vi "Dashboard Main.vi"() -> ()   [LabVIEW 2013]
uses:
  <vilib>/event_ctls.llb/eventvkey.ctl
panel:
  out "Encoder Speed":dbl(graph)
  in  "Rec Mode":enum32{"Stop", "Record", "Playback"}(radio)
  out "Battery":sgl
  out "High Gear":bool
  out "Speed":dbl(knob) scale=0.0..25.0
  out "Dashboard Connected":bool
  in  "Tab Control":enum32{"Auto", "Constants", "Checklist", "Gyro"}(tab)
  in  "Autonmous To Run":string(combo)
  in  "Autonmous mode":string
  in  "Editable":bool
  in  "Reload Autonmous text file":bool
  in  "Save Auto file back to text file":bool
  in  "Reload Constants":bool
  out "Variable Names":string[](array[string])
  out "Array of Numbers":dbl[](array[numeric])
  in  "Listbox":i32(listbox)
  in  "Reset Gyro":bool
  out "gyroAngle":dbl
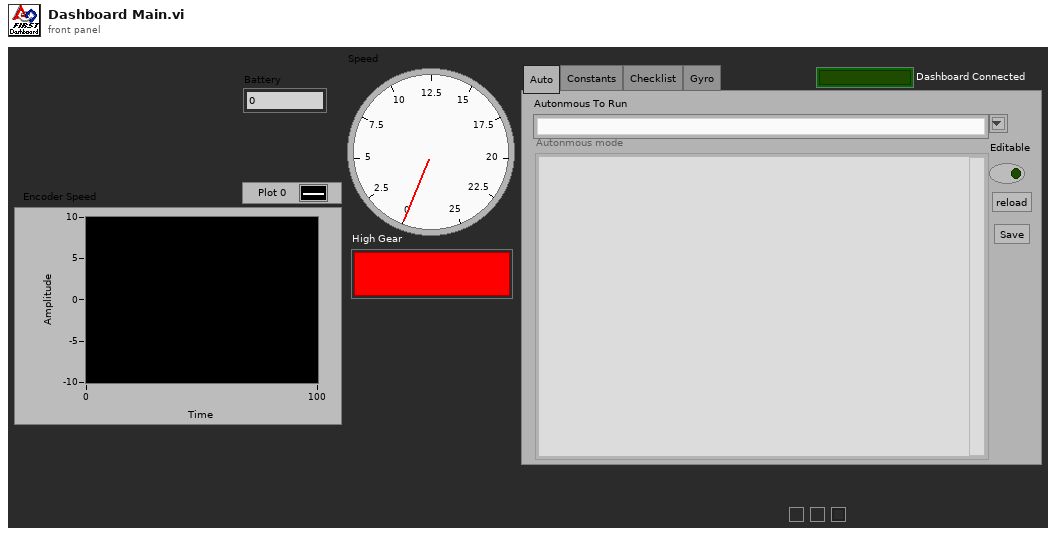
[diagram p1: front panel]
types:
  T1 = enum16{"None", "On Hover", "On Key Focus", "On Hover or Key Focus"}
  T2 = enum8{"Enabled", "Disabled", "Disabled and Grayed Out"}
  T3 = cluster{"Digital Inputs":bool[], "Digital Outputs":bool[]}
  T4 = cluster{"Competition mode":bool, "Robot Link":bool, "Autonomous":bool, "Enabled":bool, "E-Stop":bool, "Simulated":bool, "TestMode":bool, "Docked Window":bool}
  T5 = typedef "eventvkey.ctl" = enum16{"ASCII", "Enter", "Return", "Shift", "Ctrl", "Alt", "Cmd", "Opt", "Caps", "NumLock", "Clear", "Break", "Up", "Down", "Left", "Right", "Insert", "Delete", "Home", "End", "PageUp", "PageDown", "Escape", "Help", "Pause", "ScrollLock", "F1", "F2", "F3", "F4", "F5", "F6", "F7", "F8", "F9", "F10", "F11", "F12", "F13", "F14", "F15", "F16", "F17", "F18", "F19", "F20", "F21", "F22", "F23", "F24", "Play", "VolumeUp", "VolumeDown", "Mute", "Two Byte Char"}
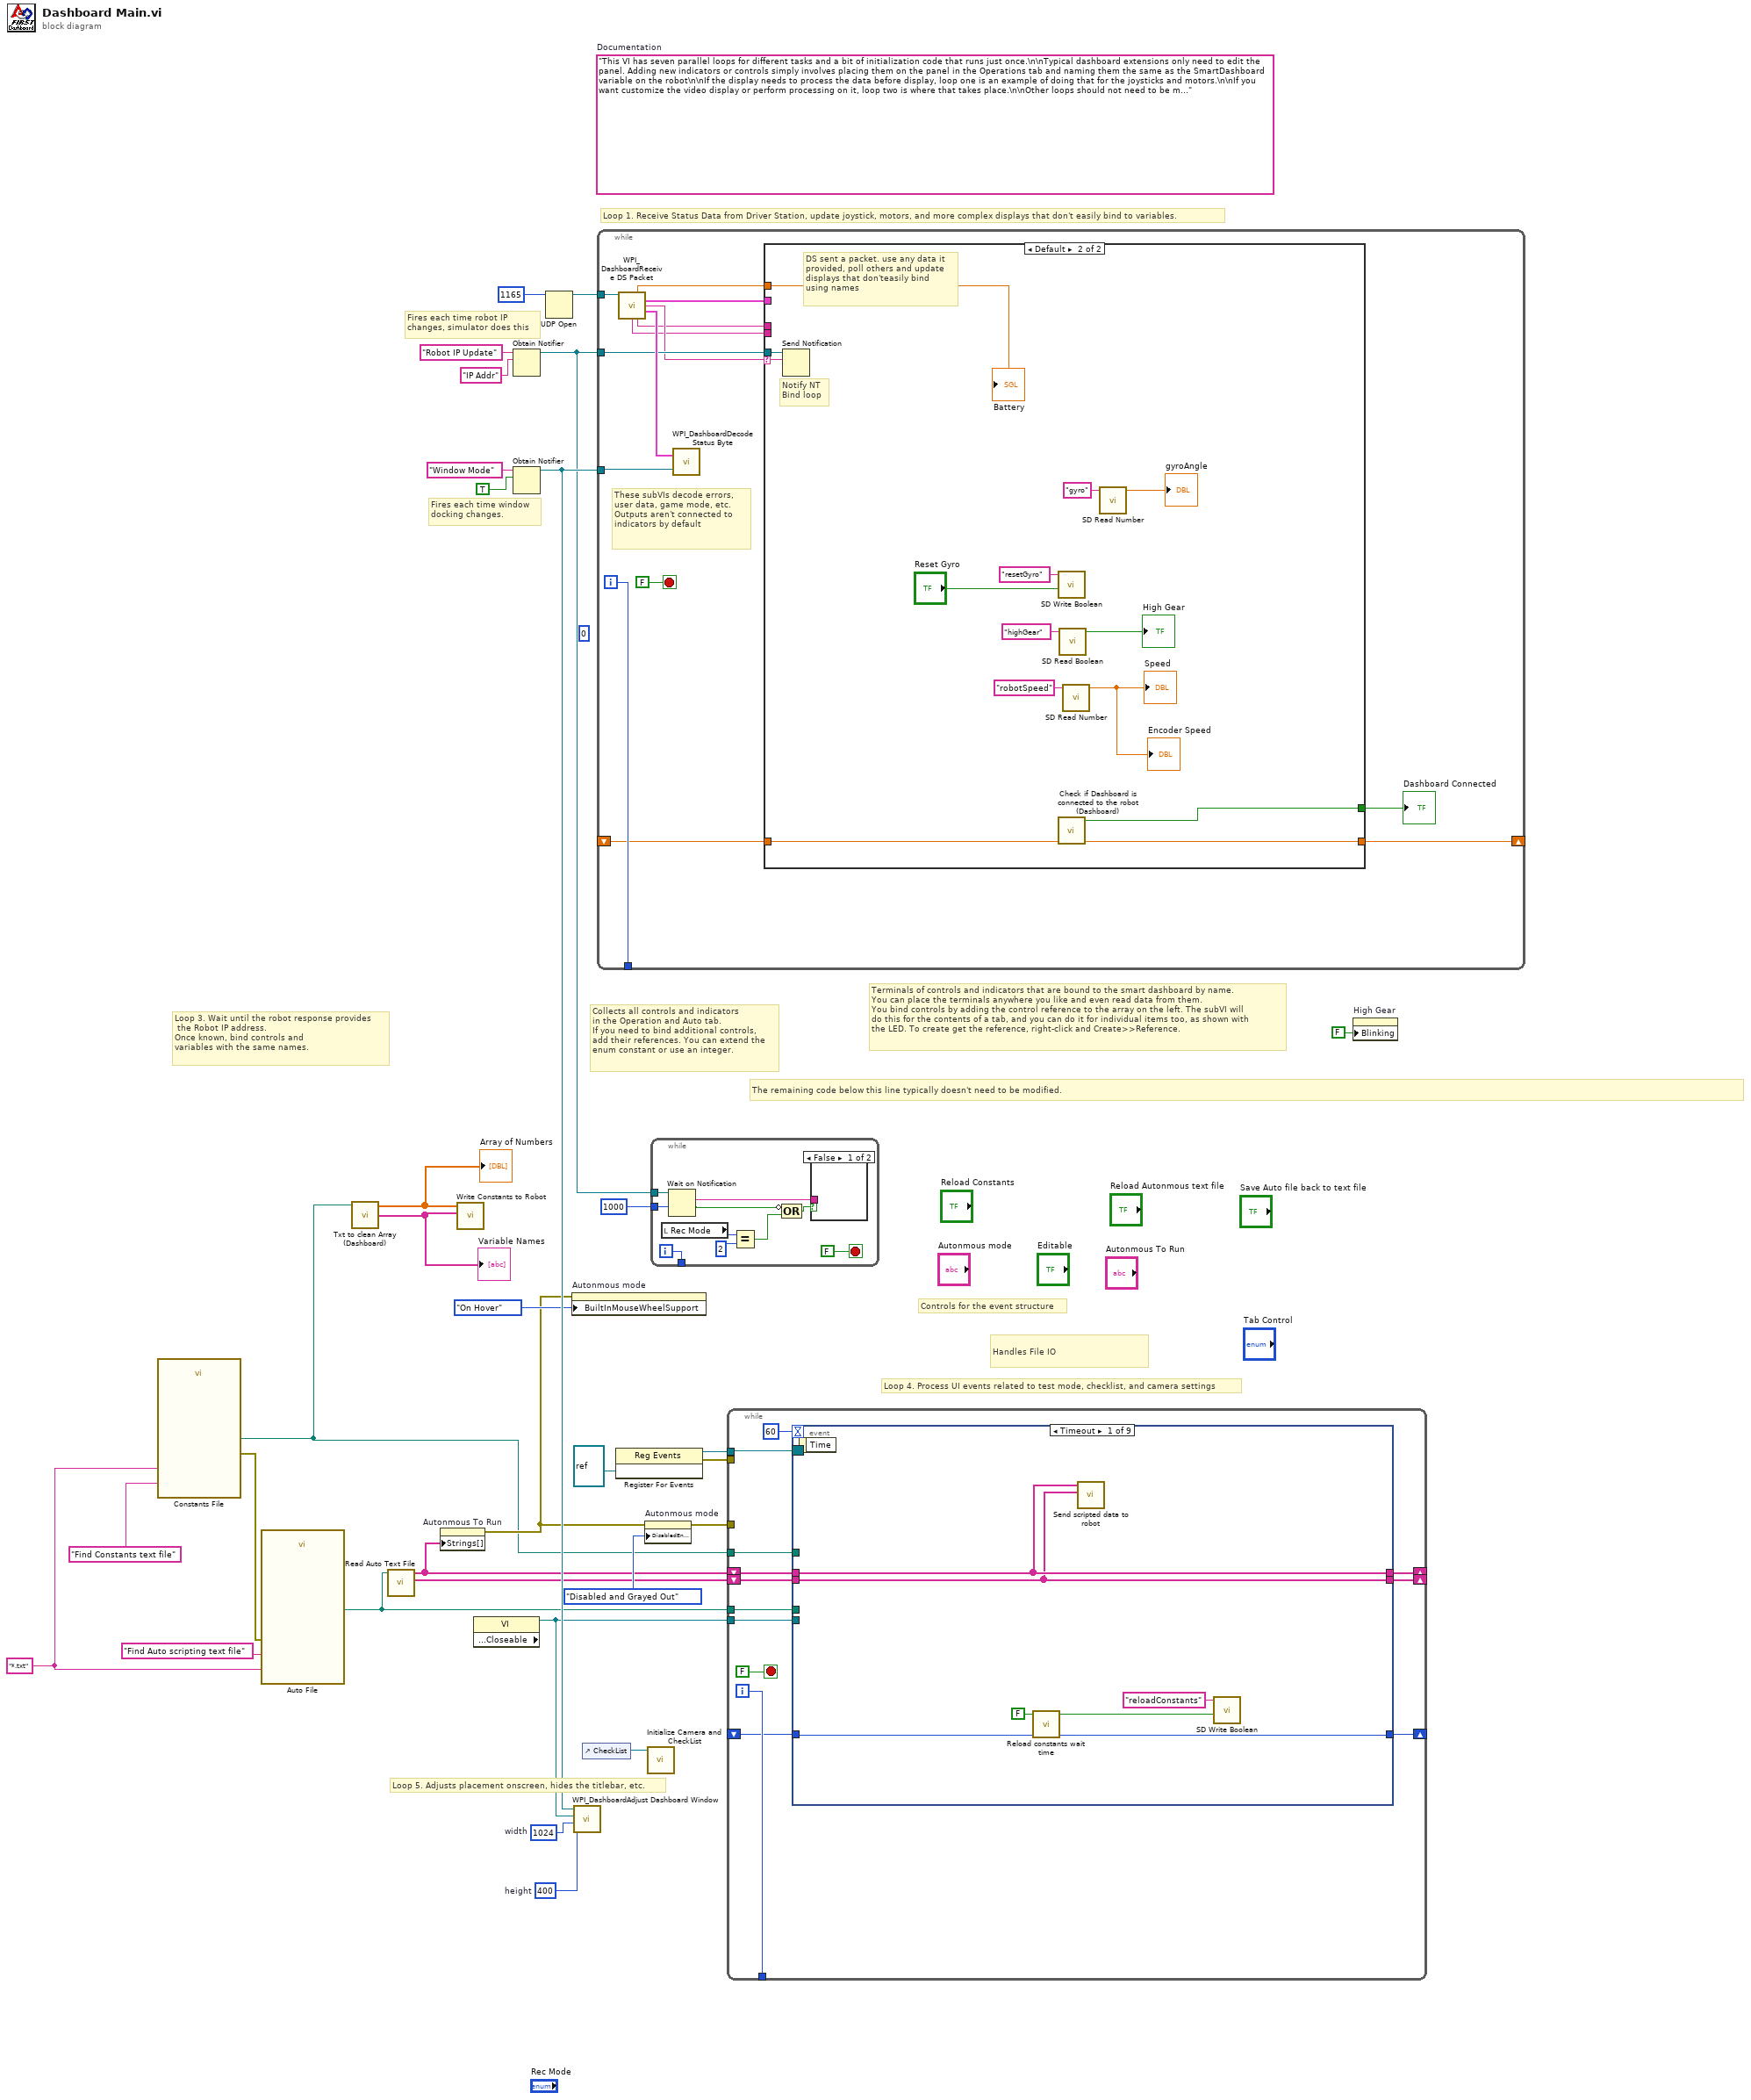
[diagram p0: block diagram]
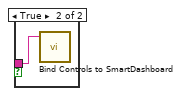
[diagram p2: hidden frame]
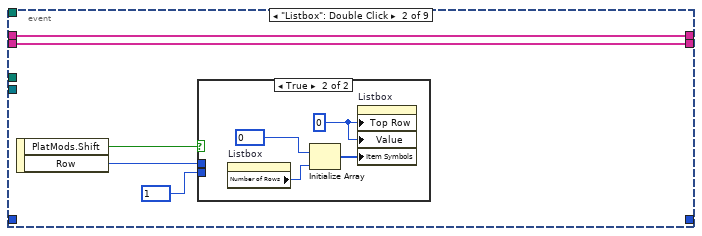
[diagram p3: hidden frame]
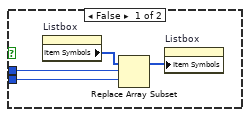
[diagram p4: hidden frame]
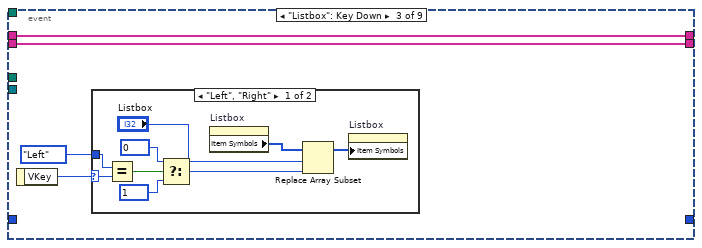
[diagram p5: hidden frame]
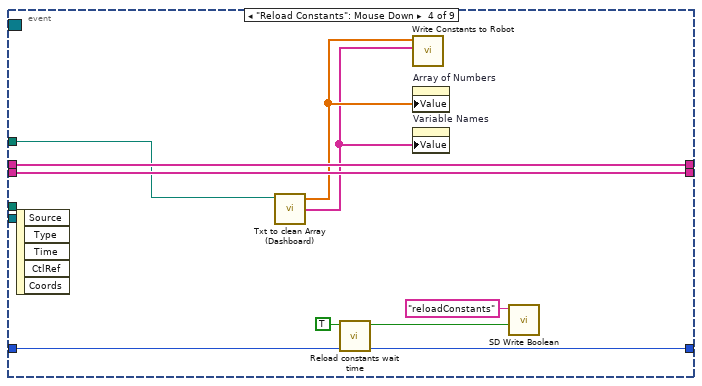
[diagram p7: hidden frame]
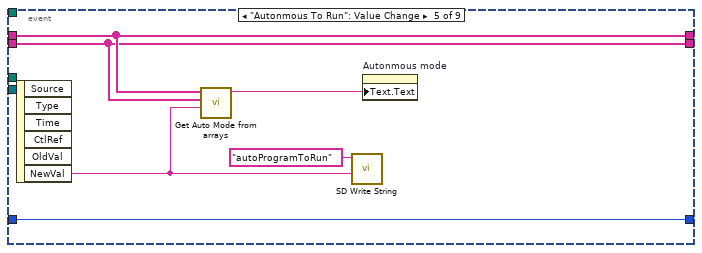
[diagram p8: hidden frame]
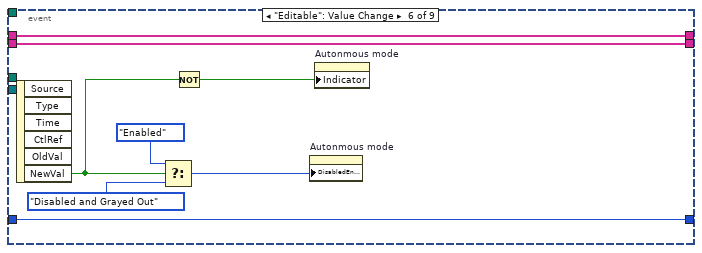
[diagram p9: hidden frame]
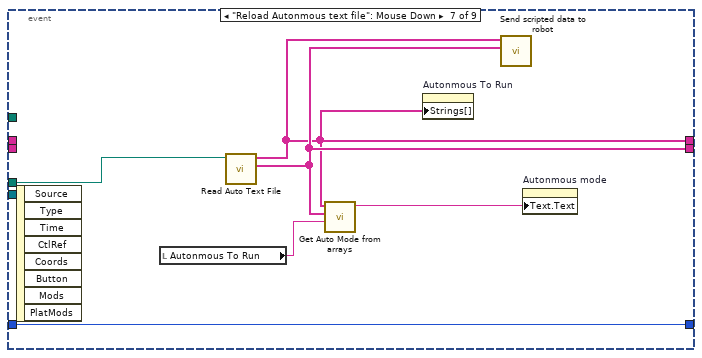
[diagram p10: hidden frame]
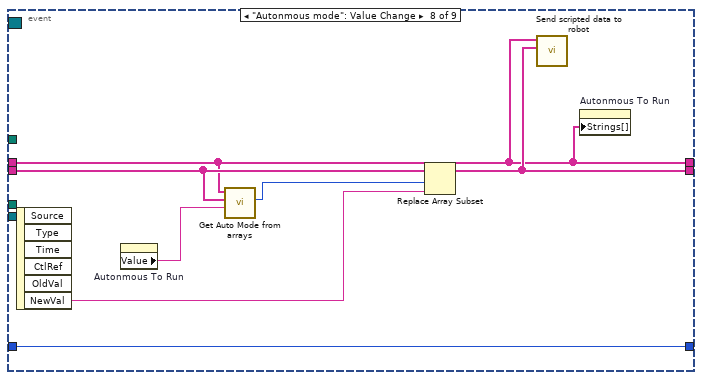
[diagram p11: hidden frame]
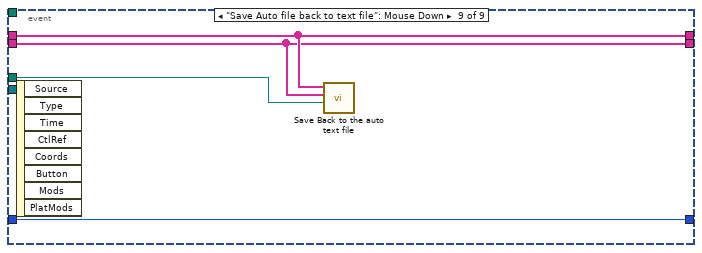
[diagram p12: hidden frame]
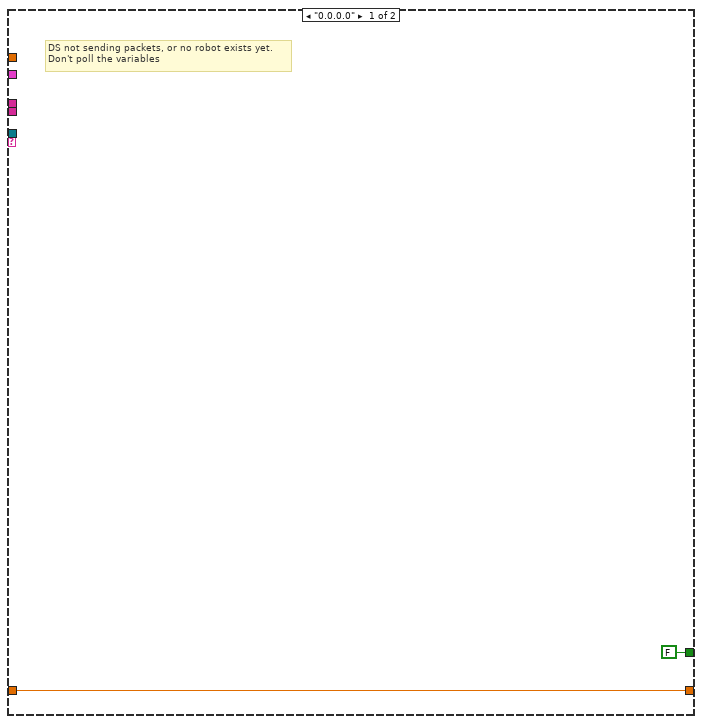
[diagram p13: hidden frame]
diagram:
  (unwired) u32 0 ("millisecond timer value out")
  w7 = "*.txt" ("pattern label")
  w21 = 400  # height
  w22 = 1024  # width
  (unwired) "This VI has seven parallel loops for different tasks and a bit of initialization code that runs just once.\n\nTypical dashboard extensions only need to edit the panel. Adding new indicators or controls simply involves placing them on the panel in the Operations tab and naming them the same as the SmartDashboard variable on the robot\n\nIf the display needs to process the data before display, loop one is an example of doing that for the joysticks and motors.\n\nIf you want customize the video display or perform processing on it, loop two is where that takes place.\n\nOther loops should not need to be modified. They are pretty standard, and document the task they perform."  # Documentation
  # "Loop 3. Wait until the robot response provides\n the Robot IP address.\nOnce known, bind controls and\nvariables with the same names."
  # "Controls for the event structure"
  # "Handles File IO"
  # "Fires each time robot IP\nchanges, simulator does this"
  # "Fires each time window\ndocking changes."
  # "Collects all controls and indicators\nin the Operation and Auto tab.\nIf you need to bind additional controls,\nadd their references. You can extend the\nenum constant or use an integer."
  # "The remaining code below this line typically doesn't need to be modified."
  # "Loop 4. Process UI events related to test mode, checklist, and camera settings"
  # "Terminals of controls and indicators that are bound to the smart dashboard by name.\nYou can place the terminals anywhere you like and even read data from them.\nYou bind controls by adding the control reference to the array on the left. The subVI will\ndo this for the contents of a tab, and you can do it for individual items too, as shown with\nthe LED. To create get the reference, right-click and Create>>Reference."
  # "Loop 5. Adjusts placement onscreen, hides the titlebar, etc."
  # "Loop 1. Receive Status Data from Driver Station, update joystick, motors, and more complex displays that don't easily bind to variables."
  n1 = call "Constants File"("prompt"="Find Constants text file", "pattern (all files)"=w7) -> ("selected path"=w10:path, "error out"=w9:errorcluster)  [unwired: 10 in, 2 out]
  n2 = call "Auto File"("prompt"="Find Auto scripting text file", "error in"=w9, "pattern (all files)"=w7) -> ("selected path"=w17:path)  [unwired: 9 in, 3 out]
  n3 = call "Txt to clean Array (Dashboard).vi"("file path"=w10) -> ("Variable Names"=w4:string[], "Array of Numbers"=w5:dbl[])  [unwired: 3 in, 1 out]
  "Array of Numbers" <- w5
  "Variable Names" <- w4
  n4 = call "Read Auto Text File.vi"("selected path"=w17) -> ("Programs"=w14:string[], "Program Name"=w15:string[])  [unwired: 8 in, 1 out]
  n5 = property on="Autonmous To Run" class="CmbBox"("Strings[]"=w15) -> (error out=w12:errorcluster)  [unwired: 2 in, 1 out]
  n6 = call "Write Constants to Robot.vi"("Variable Names"=w4, "Array of Numbers"=w5) -> ()  [unwired: 10 in]
  n7 = property class="VI" props=["Front Panel.Closeable"]() -> (reference out=w18:refnum<vi>)  [unwired: 2 in, 2 out]
  n8 = Obtain Notifier(name (unnamed)="Robot IP Update", notification data type="IP Addr" ("name (unnamed)")) -> (notifier out=w1:refnum<notifier>)  [unwired: 2 in, 2 out]
  n9 = Obtain Notifier(name (unnamed)="Window Mode", notification data type=TRUE) -> (notifier out=w20:refnum<notifier>)  [unwired: 2 in, 2 out]
  n10 = UDP Open(11:u16 1165 ("port")) -> (port=w30:refnum<k16>)  [unwired: 2 in, 4 out]
  n11 = property on="Autonmous mode" class="Str"(error in=w12, "BuiltInMouseWheelSupport"=T1."On Hover" ("Built-In Mouse Wheel Support")) -> ()  [unwired: 1 in, 2 out]
  n12 = call <vilib>:"WPI_DashboardAdjust Dashboard Window.vi"("height"=w21, "width"=w22, "reference in"=w18, "Notifier in"=w20) -> ()  [unwired: 8 in]
  n13 = control-ref of="CheckList"() -> (w19:refnum<vi>)
  n14 = while {
    tunnel: w30 -> [w43]
    tunnel: w1 -> [w40]
    tunnel: w20 -> [w42]
    tunnel: [w41] -> _
    shift-right: [w34] -> _
    shift-left: _ -> [w33]
    i -> [w41]
    stop <- FALSE stop-if-true
    # "These subVIs decode errors, user data, game mode, etc.\nOutputs aren't connected to indicators by default"
    n15 = call <vilib>:"WPI_DashboardReceive DS Packet.vi"("Recv Socket"=w43) -> ("Battery"=w35:sgl, "Driver Station"=w36:T3, "Robot IP Address"=w39:string, "Status"=w44:T4, "Low Priority User Data"=w38:string, "High Priority User Data"=w37:string)  [unwired: 1 in, 8 out]
    n16 = call <vilib>:"WPI_DashboardDecode Status Byte.vi"("Window Mode Notifier"=w42, "Status"=w44) -> ()  [unwired: 2 out]
    n17 = case shown="Default" w39 {
      selector: w39 -> [_ w60]
      tunnel: w40 -> [_ w61]
      tunnel: w38 -> [_ _]
      tunnel: w37 -> [_ _]
      tunnel: w36 -> [_ _]
      tunnel: w35 -> [_ w54]
      tunnel: [w47 w59] -> w34
      tunnel: w33 -> [w47 w58]
      tunnel: [FALSE ("Number Changing") w53] -> w32
      frame "0.0.0.0" {
        # "DS not sending packets, or no robot exists yet.\nDon't poll the variables"
      }
      frame Default {
        # "Notify NT\nBind loop"
        # "DS sent a packet. use any data it\nprovided, poll others and update\ndisplays that don'teasily bind\nusing names"
        n18 = Send Notification(notification=w60, notifier=w61) -> ()  [unwired: 1 in, 2 out]
        n19 = call <vilib>:"SD Write Boolean.vi"("Boolean"="Reset Gyro", "Name"="resetGyro") -> ()  [unwired: 8 in, 2 out]
        n20 = call "Check if Dashboard is connected to the robot (Dashboard).vi"("From shift"=w58) -> ("to shift"=w59:dbl, "Number Changing"=w53:bool)  [unwired: 9 in]
        n21 = call <vilib>:"SD Read Boolean.vi"("Name"="highGear") -> ("Boolean"=→"High Gear":bool)  [unwired: 8 in, 2 out]
        n22 = call <vilib>:"SD Read Number.vi"("Name"="robotSpeed") -> ("Numeric"=→"Speed" →"Encoder Speed":dbl)  [unwired: 8 in, 2 out]
        n23 = call <vilib>:"SD Read Number.vi"("Name"="gyro") -> ("Numeric"=→"gyroAngle":dbl)  [unwired: 8 in, 2 out]
        "Battery" <- w54
      }
    }
    "Dashboard Connected" <- w32
  }
  n24 = register-events(refnum<vi> refnum) -> (reference out=w25:refnum<event-registration>, error out=w24:errorcluster)  [unwired: 2 in]
  n25 = property on="Autonmous mode" class="Str"(error in=w12, "DisabledEnum"=T2."Disabled and Grayed Out" ("Disabled")) -> (error out=w11:errorcluster)  [unwired: 1 in, 1 out]
  n26 = call "Initialize Camera and CheckList.vi"("ListBox in"=w19) -> ()  [unwired: 11 in]
  n27 = while {
    tunnel: w1 -> [w70]
    tunnel: [w68] -> _
    tunnel: u32 1000 ("milliseconds to wait") -> [w67]
    i -> [w68]
    stop <- FALSE stop-if-true
    n28 = local read "Rec Mode"() -> (w63:enum32{"Stop", "Record", "Playback"})
    n29 = Wait on Notification(notifier=w70, timeout in ms (-1)=w67) -> (notification=w69:string, timed out?=w65:bool)  [unwired: 2 in, 2 out]
    n30 = Equal?(x=w63, y=u16 2 ("Rec Mode")) -> (x = y?=w64:bool)
    n31 = Compound Arithmetic op=OR(invert w65, w64) -> (w66:bool)
    n32 = case shown="False" w66 {
      tunnel: w69 -> [_ w72]
      frame False {
      }
      frame True {
        n33 = call <vilib>:"Bind Controls to SmartDashboard.vi"("Server IP Address"=w72) -> ()  [unwired: 11 in]
      }
    }
  }
  n34 = while {
    tunnel: [w83] -> _
    tunnel: w25 -> [w82]
    tunnel: w24 -> [_]
    tunnel: w18 -> [w81]
    tunnel: w17 -> [w80]
    tunnel: w10 -> [w79]
    shift-right: [w76] -> _
    shift-left: w15 -> [w78]
    shift-right: [w75] -> _
    shift-left: w14 -> [w77]
    tunnel: w11 -> [_]
    shift-right: [w74] -> _
    shift-left: _ -> [w73]
    i -> [w83]
    stop <- FALSE stop-if-true
    n35 = event shown="[0] Timeout" {
      selector: w82 -> [_ _ _ _ _ _ _ _ _]
      dyn-events: _ -> [_ _ _ _ _ _ _ _ _]
      timeout: u32 60 ("milliseconds to wait") -> [_ _ _ _ _ _ _ _ _]
      tunnel: w81 -> [_ _ _ _ _ _ _ _ _]
      tunnel: w80 -> [_ _ _ _ _ _ w148 _ w157]
      tunnel: w79 -> [_ _ _ w126 _ _ _ _ _]
      tunnel: w77 -> [w91 w93 w106 w127 w130 w136 _ w154 w158]
      tunnel: w78 -> [w92 w94 w107 w128 w131 w137 _ w151 w159]
      tunnel: [w92 w94 w107 w128 w131 w137 w144 w151 w159] -> w76
      tunnel: [w91 w93 w106 w127 w130 w136 w147 w152 w158] -> w75
      tunnel: [w89 _ _ w122 w129 w135 w143 w149 w156] -> w74
      tunnel: w73 -> [w90 _ _ w123 w129 w135 w143 w149 w156]
      event Timeout {
        n36 = event-data() -> ()  [unwired: 1 in, 1 out]
        n37 = call "Reload constants wait time.vi"("millisecond timer value in"=w90, "Reload Constants"=FALSE) -> ("millisecond timer value out"=w89:u32, "Tell Robot to reload constants"=w86:bool)  [unwired: 8 in]
        n38 = call "Send scripted data to robot.vi"("Programs"=w91, "Program Name"=w92) -> ()  [unwired: 10 in]
        n39 = call <vilib>:"SD Write Boolean.vi"("Boolean"=w86, "Name"="reloadConstants") -> ()  [unwired: 8 in, 2 out]
      }
      event "Listbox": Double Click {
        n40 = event-data() -> ("PlatMods.Shift"=w95:bool, "Row"=w97:i32)  [unwired: 1 in]
        n41 = case shown="True" w95 {
          tunnel: w97 -> [w101 _]
          tunnel: 1 -> [w100 _]
          frame False {
            n42 = property on="Listbox" class="LstBox (strict)"() -> ("Item Symbols"=w99:i32[])  [unwired: 2 in, 2 out]
            n43 = Replace Array Subset(array=w99, new element=w100, index=w101) -> (w98:i32[])
            n44 = property on="Listbox" class="LstBox (strict)"("Item Symbols"=w98) -> ()  [unwired: 2 in, 2 out]
          }
          frame True {
            w102 = 0 ("Top Row")
            n45 = property on="Listbox" class="LstBox (strict)"() -> ("Number of Rows"=w104:u32)  [unwired: 2 in, 2 out]
            n46 = Initialize Array(0, w104) -> (w103:i32[])
            n47 = property on="Listbox" class="LstBox (strict)"("Top Row"=w102, "Value"=w102, "Item Symbols"=w103) -> ()  [unwired: 2 in, 2 out]
          }
        }
      }
      event "Listbox": Key Down {
        n48 = event-data() -> ("VKey"=w109:T5)  [unwired: 1 in]
        n49 = case shown="\"Left\", \"Right\"" w109 {
          selector: w109 -> [w114 _]
          tunnel: eventvkey."Left" ("VKey") -> [w112 _]
          frame "Left", "Right" {
            n50 = Equal?(x=w112, y=w114) -> (x = y?=w113:bool)
            n51 = Select(t=0, s=w113, f=1) -> (s? t:f=w115:i32)
            n52 = property on="Listbox" class="LstBox (strict)"() -> ("Item Symbols"=w118:i32[])  [unwired: 2 in, 2 out]
            n53 = Replace Array Subset(array=w118, new element=w115, index="Listbox") -> (w117:i32[])
            n54 = property on="Listbox" class="LstBox (strict)"("Item Symbols"=w117) -> ()  [unwired: 2 in, 2 out]
          }
          frame Default {
          }
        }
      }
      event "Reload Constants": Mouse Down {
        n55 = event-data() -> ()  [unwired: 1 in, 5 out]
        n56 = call "Txt to clean Array (Dashboard).vi"("file path"=w126) -> ("Variable Names"=w124:string[], "Array of Numbers"=w125:dbl[])  [unwired: 3 in, 1 out]
        n57 = call "Reload constants wait time.vi"("millisecond timer value in"=w123, "Reload Constants"=TRUE) -> ("millisecond timer value out"=w122:u32, "Tell Robot to reload constants"=w119:bool)  [unwired: 8 in]
        n58 = call "Write Constants to Robot.vi"("Variable Names"=w124, "Array of Numbers"=w125) -> ()  [unwired: 10 in]
        n59 = property on="Array of Numbers" class="Arr (strict)"("Value"=w125) -> ()  [unwired: 2 in, 2 out]
        n60 = property on="Variable Names" class="Arr (strict)"("Value"=w124) -> ()  [unwired: 2 in, 2 out]
        n61 = call <vilib>:"SD Write Boolean.vi"("Boolean"=w119, "Name"="reloadConstants") -> ()  [unwired: 8 in, 2 out]
      }
      event "Autonmous To Run": Value Change {
        n62 = event-data() -> ("NewVal"=w133:string)  [unwired: 1 in, 5 out]
        n63 = call "Get Auto Mode from arrays.vi"("Auto Name"=w133, "Programs"=w130, "Program Name"=w131) -> ("Auto Program"=w132:string)  [unwired: 7 in, 1 out]
        n64 = call <vilib>:"SD Write String.vi"("String"=w133, "Name"="autoProgramToRun") -> ()  [unwired: 8 in, 2 out]
        n65 = property on="Autonmous mode" class="Str"("Text.Text"=w132) -> ()  [unwired: 2 in, 2 out]
      }
      event "Editable": Value Change {
        n66 = event-data() -> ("NewVal"=w139:bool)  [unwired: 1 in, 5 out]
        n67 = Select(t=T2."Enabled" ("Disabled"), s=w139, f=T2."Disabled and Grayed Out" ("Disabled")) -> (s? t:f=w140:T2)
        n68 = Not(x=w139) -> (.not. x?=w138:bool)
        n69 = property on="Autonmous mode" class="Str"("DisabledEnum"=w140) -> ()  [unwired: 2 in, 2 out]
        n70 = property on="Autonmous mode" class="Str"("Indicator"=w138) -> ()  [unwired: 2 in, 2 out]
      }
      event "Reload Autonmous text file": Mouse Down {
        n71 = event-data() -> ()  [unwired: 1 in, 8 out]
        n72 = local read "Autonmous To Run"() -> (w146:string)
        n73 = call "Read Auto Text File.vi"("selected path"=w148) -> ("Programs"=w147:string[], "Program Name"=w144:string[])  [unwired: 8 in, 1 out]
        n74 = call "Get Auto Mode from arrays.vi"("Auto Name"=w146, "Programs"=w147, "Program Name"=w144) -> ("Auto Program"=w145:string)  [unwired: 7 in, 1 out]
        n75 = property on="Autonmous To Run" class="CmbBox"("Strings[]"=w144) -> ()  [unwired: 2 in, 2 out]
        n76 = call "Send scripted data to robot.vi"("Programs"=w147, "Program Name"=w144) -> ()  [unwired: 10 in]
        n77 = property on="Autonmous mode" class="Str"("Text.Text"=w145) -> ()  [unwired: 2 in, 2 out]
      }
      event "Autonmous mode": Value Change {
        n78 = event-data() -> ("NewVal"=w150:string)  [unwired: 1 in, 5 out]
        n79 = property on="Autonmous To Run" class="CmbBox"() -> ("Value"=w155:string)  [unwired: 2 in, 2 out]
        n80 = call "Get Auto Mode from arrays.vi"("Auto Name"=w155, "Programs"=w154, "Program Name"=w151) -> ("index"=w153:i32)  [unwired: 7 in, 1 out]
        n81 = Replace Array Subset(array=w154, new element=w150, index=w153) -> (w152:string[])
        n82 = call "Send scripted data to robot.vi"("Programs"=w152, "Program Name"=w151) -> ()  [unwired: 10 in]
        n83 = property on="Autonmous To Run" class="CmbBox"("Strings[]"=w151) -> ()  [unwired: 2 in, 2 out]
      }
      event "Save Auto file back to text file": Mouse Down {
        n84 = event-data() -> ()  [unwired: 1 in, 8 out]
        n85 = call "Save Back to the auto text file.vi"("Path"=w157, "Programs"=w158, "Program Name"=w159) -> ()  [unwired: 9 in]
      }
    }
  }
  n86 = property on="High Gear" class="Bool (strict)"("Blinking"=FALSE) -> ()  [unwired: 2 in, 2 out]
